vi "Save Experiment File.vi"(7 "Confirm Replace File? (T)":bool=TRUE, 8 "error in (no error)":errorcluster, 10 "Experiment File Full Path":path, 11 "Experiment File Cluster":T1) -> (0 "error out":errorcluster, 1 "cancelled":bool, 2 "JSON string":string, 3 "Experiment File Cluster (duplicate)":T1)   [LabVIEW 2020, in "Experiment File.lvlib"]
uses:
  Experiment File.lvlib
  Experiment File Cluster.ctl
  Plugin Servers/Controller/Minimal Controller Cluster.ctl
  Plugin Servers/Parameter to Hardware Map/Minimal Map.ctl
  Plugin Servers/Parameter to Hardware Map/Minimal Pair Cluster.ctl
  Plugin Servers/Controller/Generic Plugin.lvclass
  Plugin Servers/Parameter to Hardware Map/Parameter to Hardware Map.lvclass
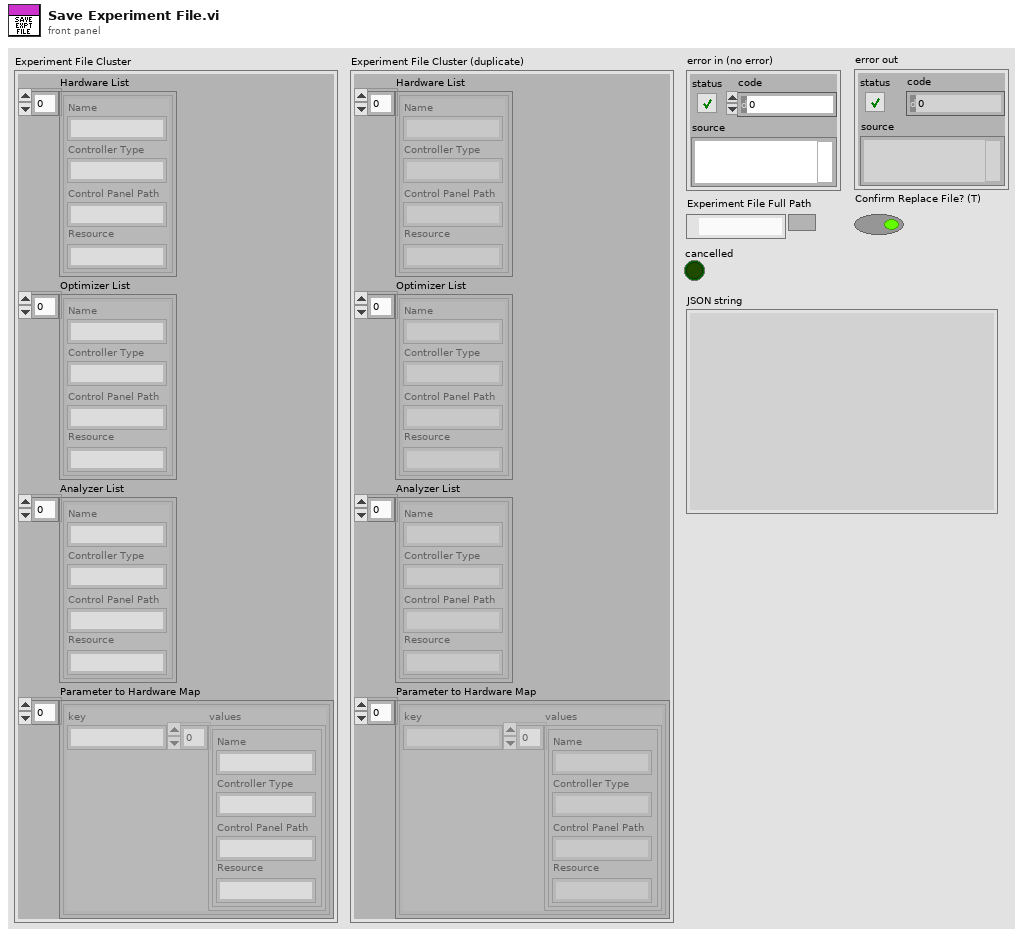
[diagram p1: front panel]
types:
  T1 = typedef "Experiment File.lvlib/Experiment File Cluster.ctl" = cluster{"Hardware List":T2[], "Optimizer List":T2[], "Analyzer List":T2[], "Parameter to Hardware Map":T3}
  T2 = typedef "Generic Plugin.lvclass/Minimal Controller Cluster.ctl" = cluster{"Name":string, "Controller Type":string, "Control Panel Path":string, "Resource":string}
  T3 = typedef "Parameter to Hardware Map.lvclass/Minimal Map.ctl" = T4[]
  T4 = typedef "Parameter to Hardware Map.lvclass/Minimal Pair Cluster.ctl" = cluster{"key":string, "values":T2[]}
  T5 = enum16{"open", "replace", "create", "open or create", "replace or create", "replace or create with confirmation"}
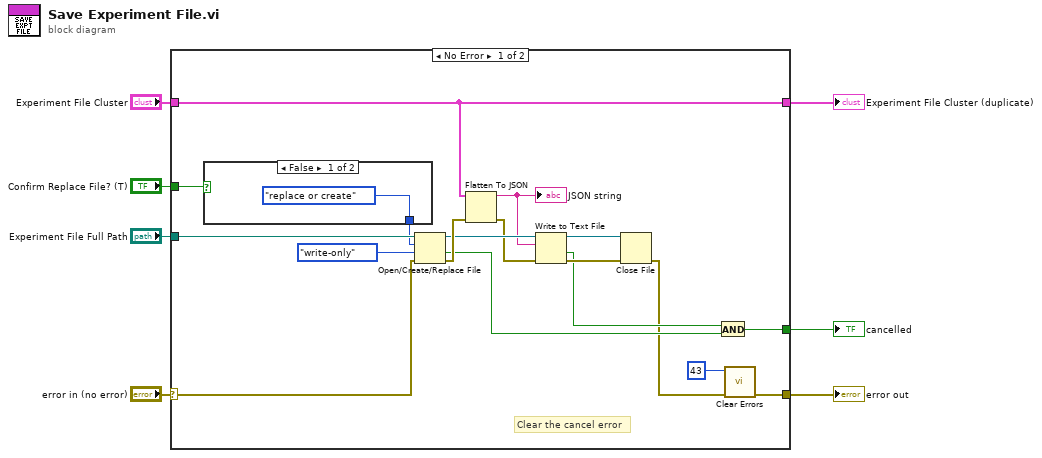
[diagram p0: block diagram]
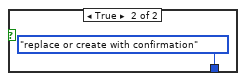
[diagram p2: hidden frame]
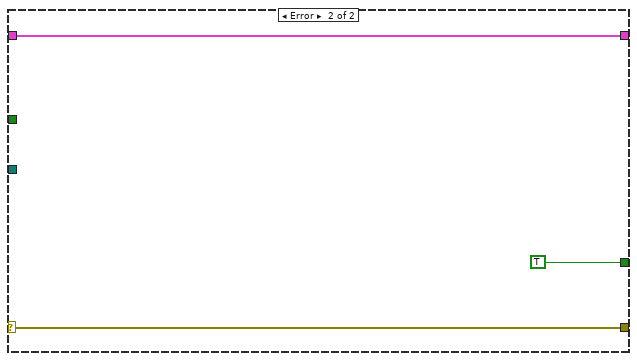
[diagram p3: hidden frame]
diagram:
  n1 = case shown="No Error" "error in (no error)" {
    selector: "error in (no error)" -> [w22 w29]
    tunnel: [w10 w29] -> w6
    tunnel: "Experiment File Cluster" -> [w16 w30]
    tunnel: [w16 w30] -> w4
    tunnel: "Experiment File Full Path" -> [w25 _]
    tunnel: [w12 TRUE] -> w2
    tunnel: "Confirm Replace File? (T)" -> [w8 _]
    frame No Error {
      # "Clear the cancel error"
      n2 = case shown="False" w8 {
        tunnel: [T5."replace or create" ("operation (0:open)") T5."replace or create with confirmation" ("operation (0:open)")] -> w24
        frame False {
        }
        frame True {
        }
      }
      n3 = Open/Create/Replace File(file path (use dialog)=w25, error in=w22, operation (0:open)=w24, access (0:read/write)=enum16{"read/write", "read-only", "write-only"}."write-only") -> (refnum out=w20:refnum<file>, cancelled=w13:bool, error out=w21:errorcluster)  [unwired: 2 in]
      n4 = Flatten To JSON(anything=w16, error in (no error)=w21) -> (JSON string=w15:string, 11:w19:errorcluster)  [unwired: 1 in]
      "JSON string" <- w15
      n5 = Write to Text File(file (use dialog)=w20, text=w15, error in=w19) -> (refnum out=w17:refnum<file>, cancelled=w14:bool, error out=w18:errorcluster)  [unwired: 1 in]
      n6 = Close File(refnum=w17, error in=w18) -> (error out=w11:errorcluster)  [unwired: 1 out]
      n7 = And(x=w14, y=w13) -> (x .and. y?=w12:bool)
      n8 = call <vilib>:"Clear Errors.vi"("error in (no error)"=w11, "specific error code to clear (0: all)"=43) -> ("error out"=w10:errorcluster)  [unwired: 4 in, 1 out]
    }
    frame Error {
    }
  }
  "Experiment File Cluster (duplicate)" <- w4
  "error out" <- w6
  "cancelled" <- w2
